vi "Disable Last Unselected for Remove Elements Action.vi"(8 "error in":errorcluster, 11 "Tree Ref":refnum<vi>) -> (0 "error out":errorcluster, 2 "Removed Item Tag":string, 3 "Tree Ref Out":refnum<vi>)   [LabVIEW 2023]
doc: "You can't remove all element from an unbundler, so don't allow selection of last unselected element. Here if all were selected (such as by shift-click), we deselect the last element selected. If one unselected remains, we disable that item."
uses:
  <userlib>/_OpenG.lib/array/array.llb/openg_array.lvlib
panel:
  in  "Tree":string[](tree)
  # "Actually, this is the item removed from the list of items selected for removal. how's that for confusing?"
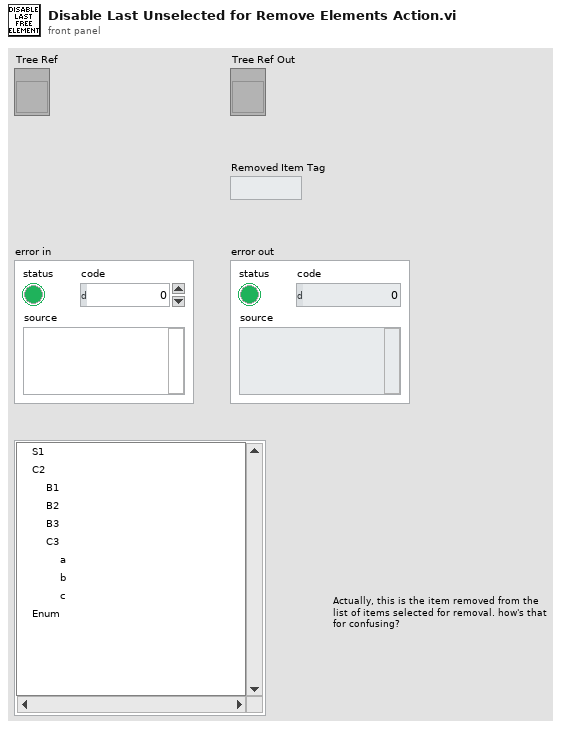
[diagram p1: front panel]
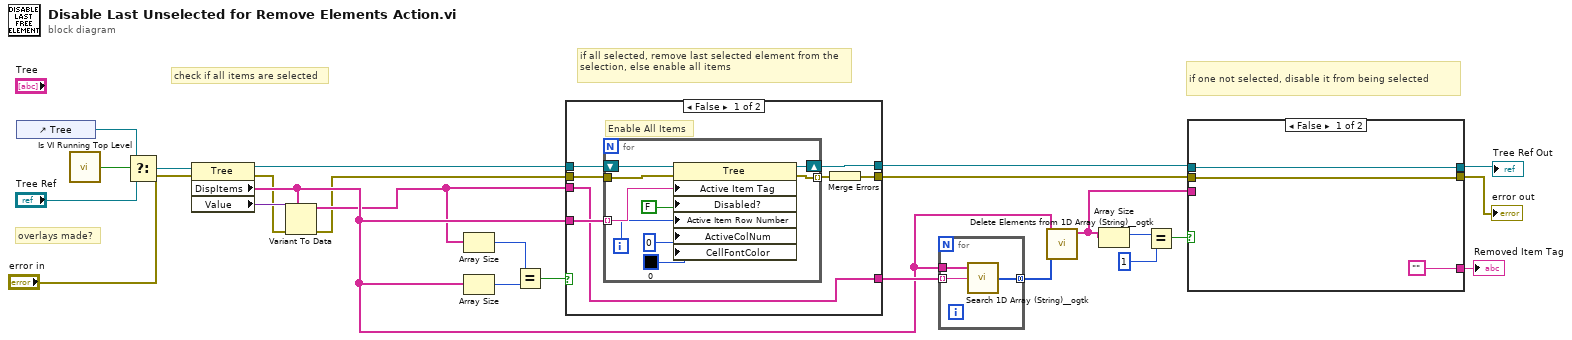
[diagram p0: block diagram]
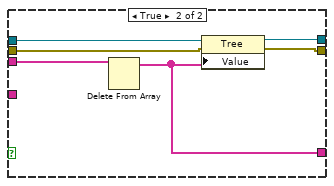
[diagram p2: hidden frame]
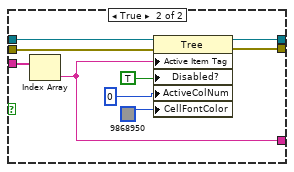
[diagram p3: hidden frame]
diagram:
  # "if one not selected, disable it from being selected"
  # "if all selected, remove last selected element from the selection, else enable all items"
  # "check if all items are selected"
  # "overlays made?"
  n1 = control-ref of="Tree"() -> (w24:refnum<vi>)
  n2 = call "Is VI Running Top Level.vi"() -> ("Top Level?"=w25:bool)  [unwired: 5 in]
  n3 = Select(t=w24, s=w25, f="Tree Ref") -> (s? t:f=w22:refnum<vi>)
  n4 = property class="Tree"(reference=w22, error in="error in") -> (reference out=w18:refnum<vi>, error out=w6:errorcluster, "DispItems"=w8:string[], "Value"=w9:variant)
  n5 = Variant To Data(error in=w6, type=w8, Variant=w9) -> (data=w7:string[], error out=w5:errorcluster)
  n6 = Array Size(array=w7) -> (size(s)=w19:i32)
  n7 = Array Size(array=w8) -> (size(s)=w20:i32)
  n8 = Equal?(x=w19, y=w20) -> (x = y?=w21:bool)
  n9 = case shown="False" w21 {
    tunnel: w18 -> [w32 w47]
    tunnel: w7 -> [w29 w46]
    tunnel: [w31 w45] -> w12
    tunnel: [w29 w44] -> w11
    tunnel: w8 -> [w30 _]
    tunnel: w5 -> [w28 w43]
    tunnel: [w26 w42] -> w4
    frame False {
      # "Enable All Items"
      n10 = for {
        shift-right: [w40] -> w31
        shift-left: w32 -> [w41]
        tunnel: w30 -> [w39] mode=indexing
        tunnel: w28 -> [w34]
        tunnel: [w33] -> w27 mode=indexing
        i -> [w35]
        n11 = property class="Tree"(reference=w41, error in=w34, "Active Item Tag"=w39, "Disabled?"=FALSE, "Active Item Row Number"=w35, "ActiveColNum"=0, "CellFontColor"=u32 0) -> (reference out=w40:refnum<vi>, error out=w33:errorcluster)
      }
      n12 = Merge Errors(w27) -> (w26:errorcluster)
    }
    frame True {
      n13 = Delete From Array(array=w46) -> (array with subset deleted=w44:string[])  [unwired: 2 in, 1 out]
      n14 = property class="Tree"(reference=w47, error in=w43, "Value"=w44) -> (reference out=w45:refnum<vi>, error out=w42:errorcluster)
    }
  }
  n15 = for {
    tunnel: [w50] -> w17 mode=concatenating
    tunnel: w11 -> [w49] mode=indexing
    tunnel: w8 -> [w48]
    n16 = call <userlib>:"Search 1D Array (String)__ogtk.vi"("Array"=w48, "Element Data"=w49) -> ("Indices of Elements"=w50:i32[])  [unwired: 7 in]
  }
  n17 = call <userlib>:"Delete Elements from 1D Array (String)__ogtk.vi"("indices"=w17, "array"=w8) -> ("array w/ subset deleted"=w13:string[])  [unwired: 8 in, 1 out]
  n18 = Array Size(array=w13) -> (size(s)=w16:i32)
  n19 = Equal?(x=w16, y=1) -> (x = y?=w14:bool)
  n20 = case shown="False" w14 {
    tunnel: w12 -> [w53 w62]
    tunnel: w13 -> [_ w61]
    tunnel: [w53 w59] -> w10
    tunnel: [w52 w56] -> w3
    tunnel: w4 -> [w52 w55]
    tunnel: ["" w54] -> w1
    frame False {
    }
    frame True {
      n21 = Index Array(array=w61) -> (element=w54:string)  [unwired: 1 in]
      n22 = property class="Tree"(reference=w62, error in=w55, "Active Item Tag"=w54, "Disabled?"=TRUE, "ActiveColNum"=0, "CellFontColor"=u32 9868950) -> (reference out=w59:refnum<vi>, error out=w56:errorcluster)
    }
  }
  "Tree Ref Out" <- w10
  "error out" <- w3
  "Removed Item Tag" <- w1
